vi "MTS_GetNextFileName.vi"(8 "error in (no error)":errorcluster, 9 "File Type":string="pt3", 10 "Measurement Type":string, 11 "Workspace":path) -> (0 "error out":errorcluster, 3 "Next File Name":path)   [LabVIEW 2013]
doc: "This vi returns the full path to the next file in the directory specified by the Save Path, User Name and the current system time in the format:\n\nSave Path\\User Name\\yyyymmdd\\0000.tcd"
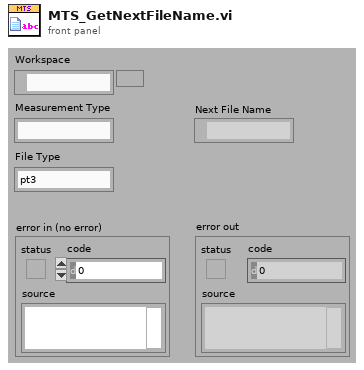
[diagram p1: front panel]
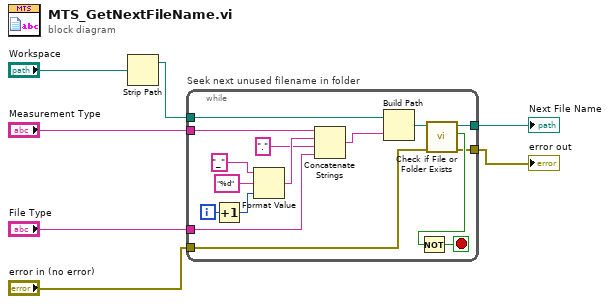
[diagram p0: block diagram]
diagram:
  n1 = Strip Path(path="Workspace") -> (stripped path=w3:path)  [unwired: 1 out]
  n2 = while "Seek next unused filename in folder" {
    tunnel: w3 -> [w23]
    tunnel: [w18] -> w7
    tunnel: "error in (no error)" -> [w17]
    tunnel: [w16] -> w6
    tunnel: "Measurement Type" -> [w11]
    tunnel: "File Type" -> [w8]
    i -> [w13]
    stop <- w20 stop-if-true
    n3 = Increment(x=w13) -> (x+1=w12:i32)
    n4 = Format Value(string ("")="_", format string="%d", value (0)=w12) -> (output string=w14:string)
    n5 = Concatenate Strings(w11, w14, "." ("string"), w8) -> (w22:string)
    n6 = Build Path(base path=w23, name or relative path=w22) -> (appended path=w21:path)
    n7 = call <vilib>:"Check if File or Folder Exists.vi"("error in (no error)"=w17, "path"=w21) -> ("error out"=w16:errorcluster, "file or folder exists?"=w19:bool, "dup path"=w18:path)  [unwired: 7 in]
    n8 = Not(x=w19) -> (.not. x?=w20:bool)
  }
  "Next File Name" <- w7
  "error out" <- w6
